vi "Read Range.vi"(8 "error in (no error)":errorcluster, 11 "Ranging Sensor in":refnum<class "Ranging Sensor.lvclass">) -> (0 "error out":errorcluster, 2 "Range":dbl, 3 "Ranging Sensor out":refnum<class "Ranging Sensor.lvclass">)   [LabVIEW 2020, in "CTI-Peripheral.lvlib" / "Ranging Sensor.lvclass"]
uses:
  Ranging Sensor.lvclass
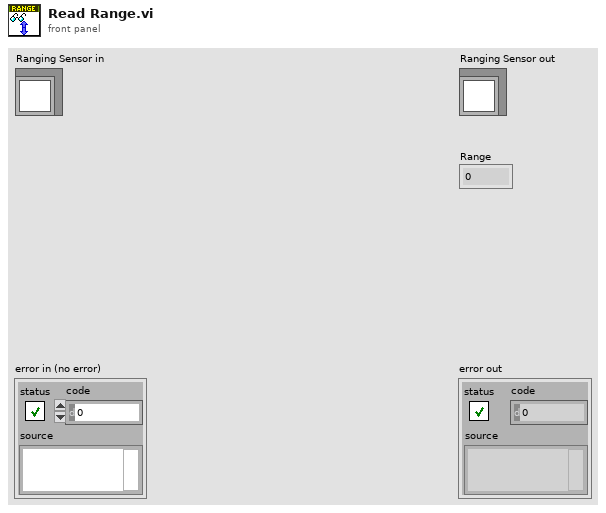
[diagram p1: front panel]
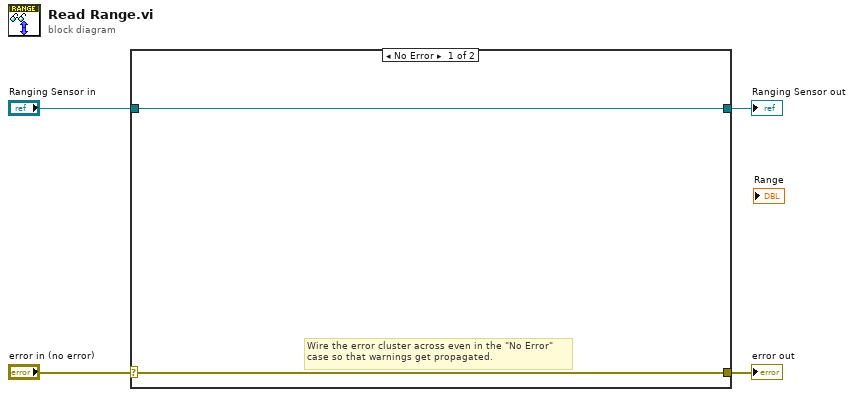
[diagram p0: block diagram]
diagram:
  n1 = case shown="No Error" "error in (no error)" {
    selector: "error in (no error)" -> [w5 w8]
    tunnel: [w5 w8] -> w3
    tunnel: [w6 w7] -> w1
    tunnel: "Ranging Sensor in" -> [w6 w7]
    frame No Error {
      # "Wire the error cluster across even in the \"No Error\"\ncase so that warnings get propagated."
    }
    frame Error {
    }
  }
  "error out" <- w3
  "Ranging Sensor out" <- w1
